vi "ProgBar_Send.vi"(5 "Stop":bool, 6 "State Info(Optional)":string, 7 "Max Number Of Iterations":i32, 8 "error in":errorcluster, 9 "Current Iteration":i32, 10 "ProgBar Label":string, 11 "ProgBar Que Name":string) -> (0 "error out":errorcluster, 1 "Cancelled?":bool)   [LabVIEW 2020]
doc: "Shows the information about the loop real time."
uses:
  controls/ProgBar_Msg.ctl
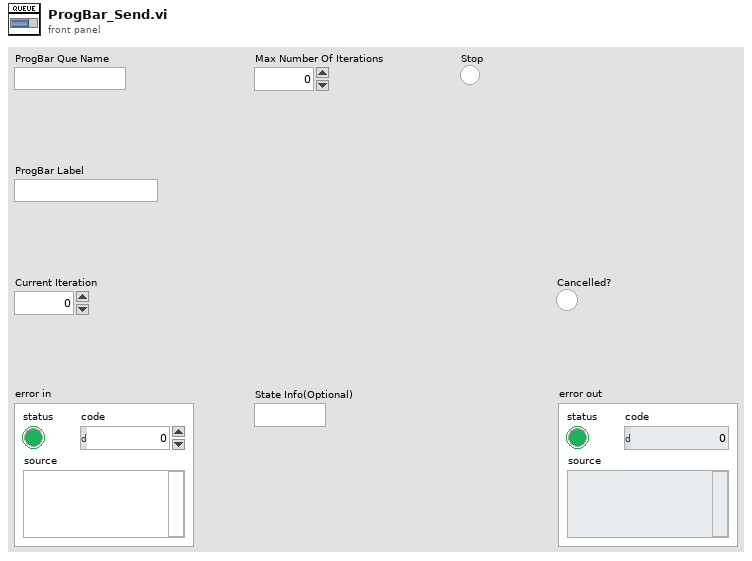
[diagram p1: front panel]
types:
  T1 = typedef "ProgBar_Msg.ctl" = cluster{"Que_Name":string, "Label":string, "Max Number of Iterations":i32, "Current Iteration ":i32, "State Info(Optional)":string, "Stop":bool}
  T2 = enum32{"Invalid", "Standard", "Closed", "Hidden", "Minimized", "Maximized"}
  T3 = enum32{"Bad", "Idle", "Run top level", "Running"}
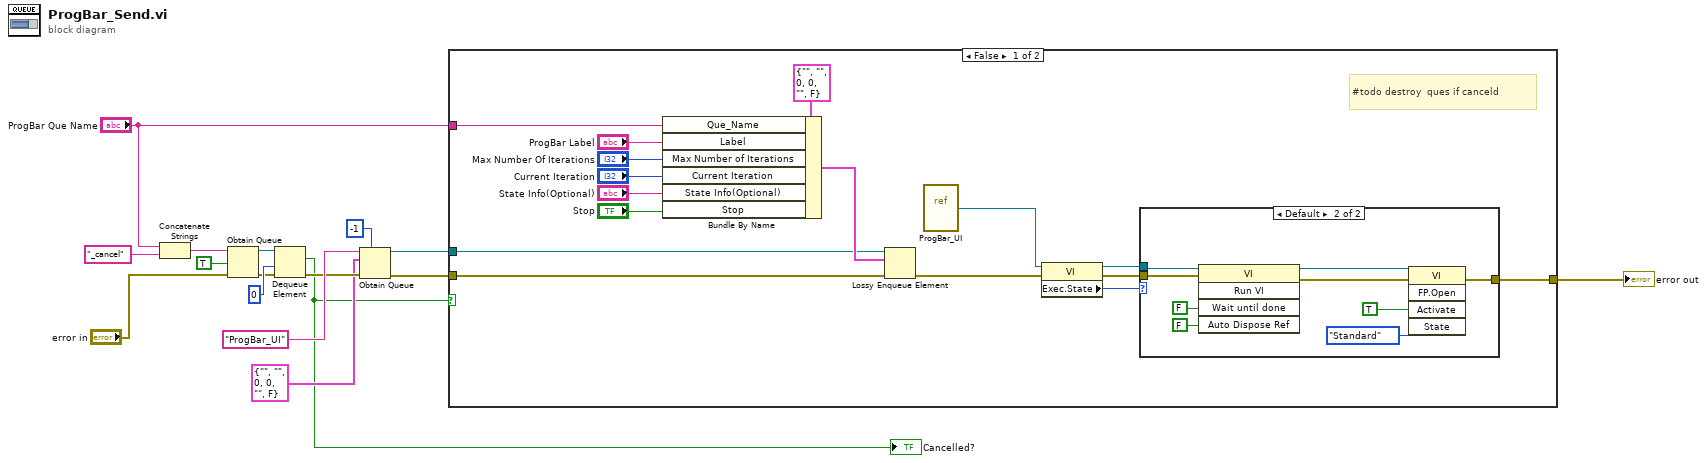
[diagram p0: block diagram]
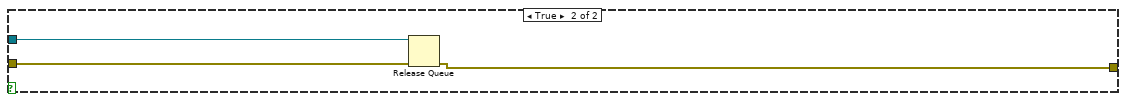
[diagram p3: hidden frame]
diagram:
  n1 = Concatenate Strings("ProgBar Que Name", "_cancel" ("string")) -> (w15:string)
  n2 = Obtain Queue(name (unnamed)=w15, element data type=TRUE, error in (no error)="error in") -> (queue out=w13:refnum<queue>, error out=w11:errorcluster)  [unwired: 2 in, 1 out]
  n3 = Dequeue Element(queue=w13, timeout in ms (-1)=0, error in (no error)=w11) -> (element=w1:bool, error out=w8:errorcluster)  [unwired: 2 out]
  "Cancelled?" <- w1
  n4 = Obtain Queue(max queue size (-1, unlimited)=-1, name (unnamed)="ProgBar_UI", element data type=T1 {"Que_Name"="", "Label"="", "Max Number of Iterations"=0, "Current Iteration "=0, "State Info(Optional)"="", "Stop"=FALSE} ("Cluster"), error in (no error)=w8) -> (queue out=w7:refnum<queue>, error out=w6:errorcluster)  [unwired: 1 in, 1 out]
  n5 = case shown="False" w1 {
    tunnel: "ProgBar Que Name" -> [w27 _]
    tunnel: w7 -> [w26 w45]
    tunnel: w6 -> [w25 w44]
    tunnel: [w19 w43] -> w2
    frame False {
      # "#todo destroy  ques if canceld"
      n6 = Bundle By Name(cluster=T1 {"Que_Name"="", "Label"="", "Max Number of Iterations"=0, "Current Iteration "=0, "State Info(Optional)"="", "Stop"=FALSE} ("Cluster"), "Que_Name"=w27, "Label"="ProgBar Label", "Max Number of Iterations"="Max Number Of Iterations", "Current Iteration"="Current Iteration", "State Info(Optional)"="State Info(Optional)", "Stop"="Stop") -> (w29:T1)
      n7 = Lossy Enqueue Element(queue=w26, element=w29, error in (no error)=w25) -> (error out=w20:errorcluster)  [unwired: 3 out]
      n8 = vi-ref "ProgBar_UI.vi"() -> (w21:refnum<vi>)
      n9 = property class="VI"(reference=w21, error in=w20) -> (reference out=w32:refnum<vi>, error out=w30:errorcluster, "Exec.State"=w31:T3)
      n10 = case shown="Default" w31 {
        tunnel: w32 -> [_ w38]
        tunnel: w30 -> [w33 w37]
        tunnel: [w33 w34] -> w19
        frame "Run top level", "Running" {
        }
        frame Default {
          n11 = invoke class="VI" method="Run VI"(reference=w38, error in=w37, "Wait until done"=FALSE ("Wait Until Done"), "Auto Dispose Ref"=FALSE ("Auto Dispose Reference")) -> (reference out=w36:refnum<vi>, error out=w35:errorcluster)  [unwired: 1 in, 3 out]
          n12 = invoke class="VI" method="FP.Open"(reference=w36, error in=w35, "Activate"=TRUE ("Activate?"), "State"=T2."Standard") -> (error out=w34:errorcluster)  [unwired: 1 in, 4 out]
        }
      }
    }
    frame True {
      n13 = Release Queue(queue=w45, error in (no error)=w44) -> (error out=w43:errorcluster)  [unwired: 1 in, 2 out]
    }
  }
  "error out" <- w2
